vi "FTW-Consumer-Listener.vi"(1 "Endpoint":refnum<class "FTW-Endpoint.lvclass">, 2 "Message Handler":refnum<user-event>) -> ()   [LabVIEW 2013, in "FTW-Consumer.lvclass"]
uses:
  FTW-Consumer.lvclass
  Message/Base/FTW-Message.lvclass
  Endpoint/FTW-Endpoint.lvclass
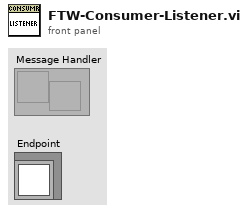
[diagram p1: front panel]
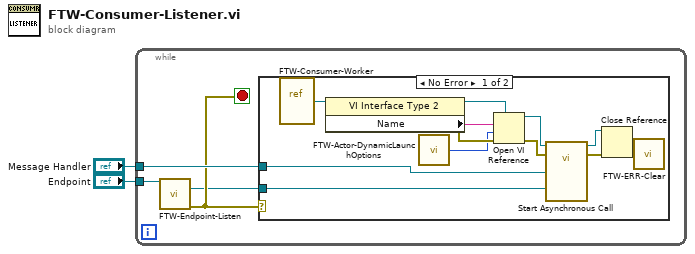
[diagram p0: block diagram]
diagram:
  n1 = while {
    tunnel: "Message Handler" -> [w5]
    tunnel: "Endpoint" -> [w6]
    stop <- w4 stop-if-true
    n2 = call-dynamic "FTW-Endpoint-Listen.vi"("FTW Endpoint"=w6) -> ("New Connection"=w3:refnum<class "FTW-Endpoint.lvclass">, "error out"=w4:errorcluster)  [unwired: 12 in, 1 out]
    n3 = case shown="No Error" w4 {
      tunnel: w5 -> [w10 _]
      tunnel: w3 -> [w9 _]
      frame No Error {
        n4 = vi-ref "FTW-Consumer-Worker.vi"() -> (w18:refnum<vi>)
        n5 = property class="VI Interface Type 2"(reference=w18) -> (reference out=w12:refnum<vi>, error out=w17:errorcluster, "Name"=w16:string)  [unwired: 1 in]
        n6 = call "FTW-Actor-DynamicLaunchOptions.vi"() -> ("Open VI Ref Options"=w15:i32)
        n7 = Open VI Reference(type specifier VI Refnum (for type only)=w12, vi path=w16, options=w15, error in (no error)=w17) -> (vi reference=w13:refnum<vi>, error out=w14:errorcluster)  [unwired: 2 in]
        n8 = call-by-ref "Start Asynchronous Call"(reference=w13, error in=w14, "Endpoint"=w9, "Message Handler"=w10) -> (reference out=w7:refnum<vi>, error out=w11:errorcluster)  [unwired: 1 in]
        n9 = Close Reference(reference=w7, error in (no error)=w11) -> (error out=w8:errorcluster)
        n10 = call "FTW-ERR-Clear.vi"("error to snuff"=w8) -> ()  [unwired: 1 out]
      }
      frame Error {
      }
    }
  }
